vi "TTLsignalactivation_171213.vi"(6 "Outside in":dbl[](array[numeric]), 8 "InputcurrentSegement":bool[](array[boolean]), 9 "Inside in":dbl[](array[numeric]), 10 "InputpriviousSegment":bool[](array[boolean]), 11 "MATCH index":i32) -> (2 "Inside out":dbl[](array[numeric]), 3 "Outside out":dbl[](array[numeric]))   [LabVIEW 2016]
uses:
  Globaltracker.vi
panel:
  in  "TTLStayingHelp":bool
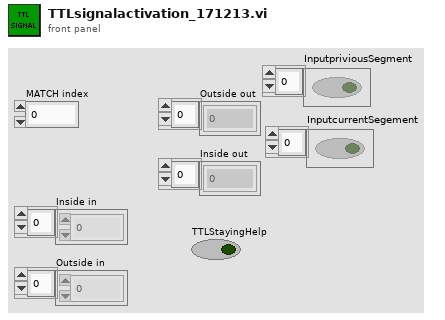
[diagram p1: front panel]
types:
  T1 = cluster{"Region number":i32, "ON/OFF":bool, "Activation type":string, "Activation critaria":i32, "Reward":i32}[]
  T2 = cluster{"Region number":i32, "ON/OFF":bool, "Activation type":string, "Activation critaria":i32, "Reward":i32}
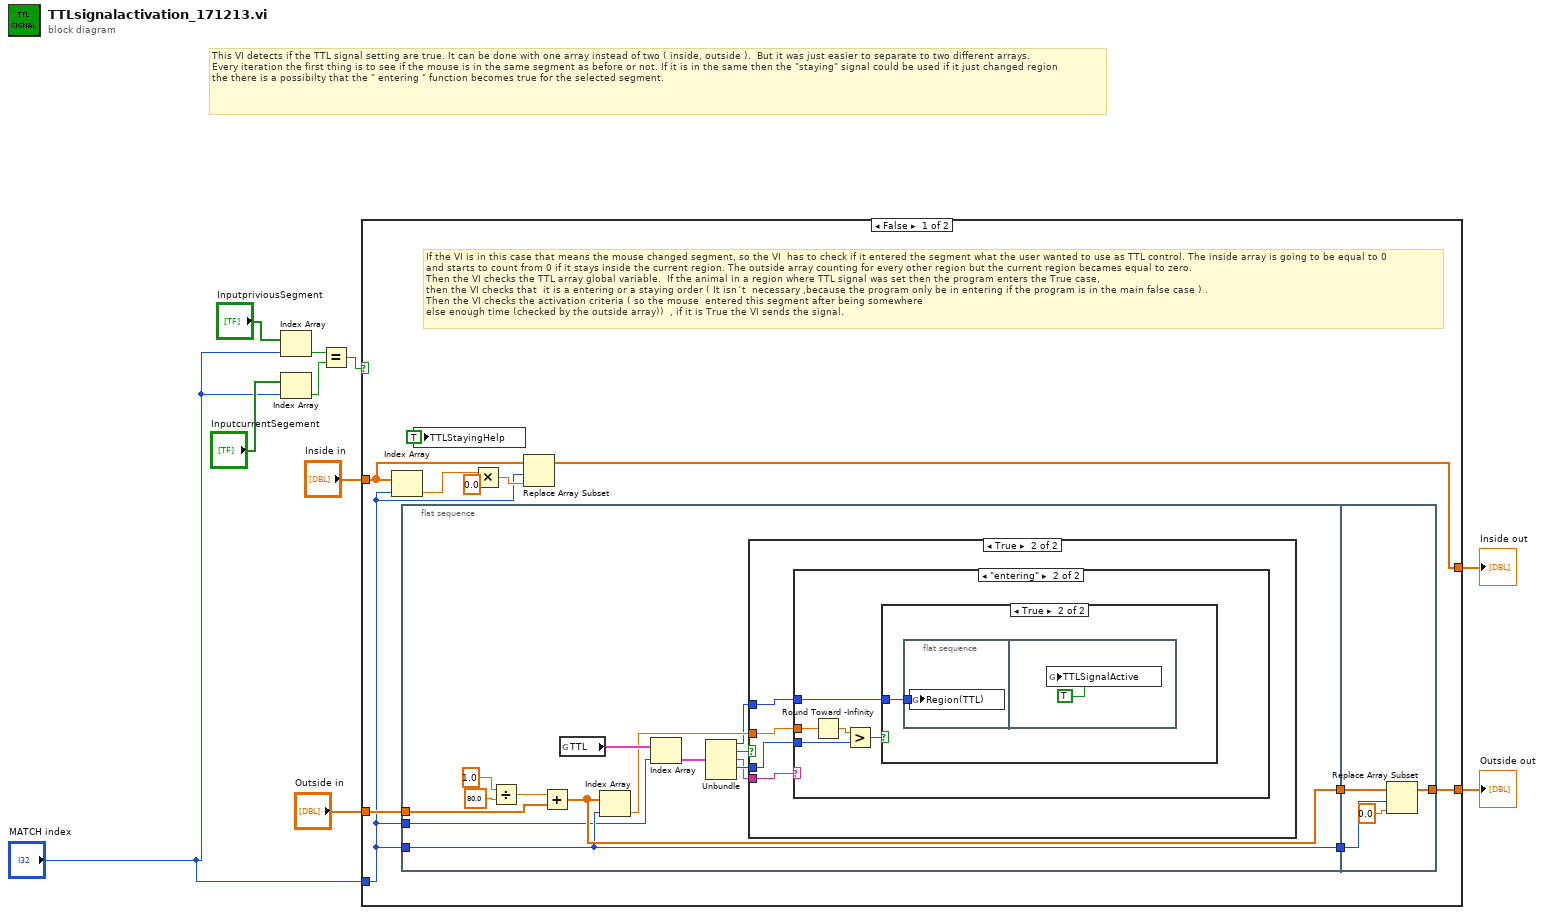
[diagram p0: block diagram]
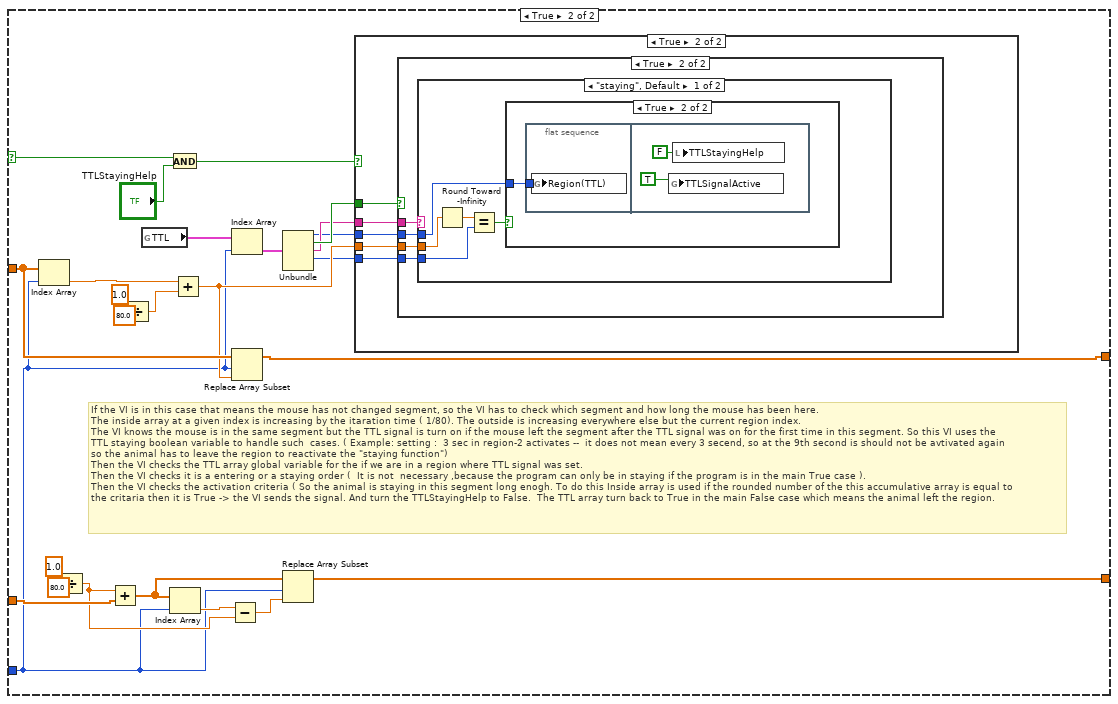
[diagram p5: hidden frame]
diagram:
  # "This VI detects if the TTL signal setting are true. It can be done with one array instead of two ( inside, outside ).  But it was just easier to separate to two different arrays.\nEvery iteration the first thing is to see if the mouse is in the same segment as before or not. If it is in the same then the \"staying\" signal could be used if it just changed region\nthe there is a possibilty that the \" entering \" function becomes true for the selected segment."
  n1 = Index Array(array="InputpriviousSegment", index="MATCH index") -> (element=w5:bool)
  n2 = Index Array(array="InputcurrentSegement", index="MATCH index") -> (element=w6:bool)
  n3 = Equal?(x=w5, y=w6) -> (x = y?=w1:bool)
  n4 = case shown="False" w1 {
    selector: w1 -> [_ w61]
    tunnel: "Inside in" -> [w19 w71]
    tunnel: [w17 w72] -> w8
    tunnel: "MATCH index" -> [w12 w57]
    tunnel: "Outside in" -> [w14 w63]
    tunnel: [w13 w64] -> w10
    frame False {
      # "If the VI is in this case that means the mouse changed segment, so the VI  has to check if it entered the segment what the user wanted to use as TTL control. The inside array is going to be equal to 0 \nand starts to count from 0 if it stays inside the current region. The outside array counting for every other region but the current region becames equal to zero. \nThen the VI checks the TTL array global variable.  If the animal in a region where TTL signal was set then the program enters the True case, \nthen the VI checks that  it is a entering or a staying order ( It isn´t  necessary ,because the program only be in entering if the program is in the main false case ) . \nThen the VI checks the activation criteria ( so the mouse  entered this segment after being somewhere \nelse enough time (checked by the outside array))  , if it is True the VI sends the signal."
      n5 = Index Array(array=w19, index=w12) -> (element=w20:dbl)
      n6 = flat-sequence {
        tunnel: w14 -> [w27]
        tunnel: w12 -> [w24]
        tunnel: [w26] -> w16
        tunnel: [w24] -> w15
        tunnel: w12 -> [w23]
        tunnel: w16 -> [w50]
        tunnel: w15 -> [w49]
        tunnel: [w51] -> w13
        frame #0 {
          n7 = Divide(x=1.0, y=80.0) -> (x/y=w28:dbl)
          n8 = Add(x=w28, y=w27) -> (x+y=w26:dbl[])
          n9 = global read "Globaltracker.vi" "TTL"() -> (w35:T1)
          n10 = Index Array(array=w26, index=w24) -> (element=w25:dbl)
          n11 = Index Array(array=w35, index=w23) -> (element=w31:T2)
          n12 = Unbundle(w31) -> ("Region number"=w22:i32, "ON/OFF"=w32:bool, "Activation type"=w33:string, "Activation critaria"=w34:i32)  [unwired: 1 out]
          n13 = case shown="True" w32 {
            tunnel: w33 -> [_ w39]
            tunnel: w34 -> [_ w38]
            tunnel: w25 -> [_ w37]
            tunnel: w22 -> [_ w36]
            frame False {
            }
            frame True {
              n14 = case shown="\"entering\"" w39 {
                tunnel: w38 -> [_ w41]
                tunnel: w37 -> [_ w42]
                tunnel: w36 -> [_ w40]
                frame "staying", Default {
                }
                frame "entering" {
                  n15 = Round Toward -Infinity(1:w42) -> (0:w43:dbl)
                  n16 = Greater?(x=w43, y=w41) -> (0:w44:bool)
                  n17 = case shown="True" w44 {
                    tunnel: w40 -> [_ w45]
                    frame False {
                    }
                    frame True {
                      n18 = flat-sequence {
                        tunnel: w45 -> [w46]
                        frame #0 {
                          n19 = global write "Globaltracker.vi" "Region(TTL)"(w46) -> ()
                        }
                        frame #1 {
                          n20 = global write "Globaltracker.vi" "TTLSignalActive"(TRUE ("Reward")) -> ()
                        }
                      }
                    }
                  }
                }
              }
            }
          }
        }
        frame #1 {
          n21 = Replace Array Subset(array=w50, new element=0.0 ("new element/subarray"), index=w49) -> (w51:dbl[])
        }
      }
      n22 = local write "TTLStayingHelp"(TRUE ("reward staying")) -> ()
      n23 = Multiply(x=w20, y=0.0) -> (x*y=w21:dbl)
      n24 = Replace Array Subset(array=w19, new element=w21, index=w12) -> (w17:dbl[])
    }
    frame True {
      # "If the VI is in this case that means the mouse has not changed segment, so the VI has to check which segment and how long the mouse has been here. \nThe inside array at a given index is increasing by the itaration time ( 1/80). The outside is increasing everywhere else but the current region index.\nThe VI knows the mouse is in the same segment but the TTL signal is turn on if the mouse left the segment after the TTL signal was on for the first time in this segment. So this VI uses the\nTTL staying boolean variable to handle such  cases. ( Example: setting :  3 sec in region-2 activates --  it does not mean every 3 secend, so at the 9th second is should not be avtivated again\nso the animal has to leave the region to reactivate the \"staying function\") \nThen the VI checks the TTL array global variable for the if we are in a region where TTL signal was set.\nThen the VI checks it is a entering or a staying order (  It is not  necessary ,because the program can only be in staying if the program is in the main True case ).\nThen the VI checks the activation criteria ( So the animal is staying in this segment long enogh. To do this Inside array is used if the rounded number of the this accumulative array is equal to \nthe critaria then it is True -> the VI sends the signal. And turn the TTLStayingHelp to False.  The TTL array turn back to True in the main False case which means the animal left the region."
      n25 = Index Array(array=w71, index=w57) -> (element=w73:dbl)
      n26 = Divide(x=1.0, y=80.0) -> (x/y=w62:dbl)
      n27 = Add(x=w62, y=w63) -> (x+y=w67:dbl[])
      n28 = Divide(x=1.0, y=80.0) -> (x/y=w74:dbl)
      n29 = global read "Globaltracker.vi" "TTL"() -> (w59:T1)
      n30 = And(x=w61, y="TTLStayingHelp") -> (x .and. y?=w60:bool)
      n31 = Index Array(array=w67, index=w57) -> (element=w68:dbl)
      n32 = Add(x=w73, y=w74) -> (x+y=w70:dbl)
      n33 = Subtract(x=w68, y=w62) -> (x-y=w69:dbl)
      n34 = Index Array(array=w59, index=w57) -> (element=w58:T2)
      n35 = Replace Array Subset(array=w71, new element=w70, index=w57) -> (w72:dbl[])
      n36 = Unbundle(w58) -> ("Region number"=w53:i32, "ON/OFF"=w56:bool, "Activation type"=w55:string, "Activation critaria"=w54:i32)  [unwired: 1 out]
      n37 = Replace Array Subset(array=w67, new element=w69, index=w57) -> (w64:dbl[])
      n38 = case shown="True" w60 {
        tunnel: w70 -> [_ w81]
        tunnel: w56 -> [_ w80]
        tunnel: w55 -> [_ w79]
        tunnel: w54 -> [_ w78]
        tunnel: w53 -> [_ w77]
        frame False {
        }
        frame True {
          n39 = case shown="True" w80 {
            tunnel: w81 -> [_ w85]
            tunnel: w79 -> [_ w84]
            tunnel: w78 -> [_ w83]
            tunnel: w77 -> [_ w82]
            frame False {
            }
            frame True {
              n40 = case shown="\"staying\", Default" w84 {
                tunnel: w85 -> [w90 _]
                tunnel: w83 -> [w87 _]
                tunnel: w82 -> [w86 _]
                frame "staying", Default {
                  n41 = Round Toward -Infinity(1:w90) -> (0:w88:dbl)
                  n42 = Equal?(x=w88, y=w87) -> (x = y?=w89:bool)
                  n43 = case shown="True" w89 {
                    tunnel: w86 -> [_ w91]
                    frame False {
                    }
                    frame True {
                      n44 = flat-sequence {
                        tunnel: w91 -> [w92]
                        frame #0 {
                          n45 = global write "Globaltracker.vi" "Region(TTL)"(w92) -> ()
                        }
                        frame #1 {
                          n46 = global write "Globaltracker.vi" "TTLSignalActive"(TRUE ("Reward")) -> ()
                          n47 = local write "TTLStayingHelp"(FALSE ("reward staying")) -> ()
                        }
                      }
                    }
                  }
                }
                frame "entering" {
                }
              }
            }
          }
        }
      }
    }
  }
  "Outside out" <- w10
  "Inside out" <- w8
